vi "AE_AllStages_Action.vi"(6 "Velocity":dbl, 7 "Abort":refnum<vi>, 8 "Positions":dbl[](array[numeric]), 9 "Axis":bool[](array[boolean]), 10 "Stage ID":string, 11 "Action":T1=enum."MVR") -> (0 "Position Out":dbl[](array[numeric]), 1 "Status":bool, 2 "Special Function Out":string)   [LabVIEW 2014]
uses:
  Controls/StageStates.ctl
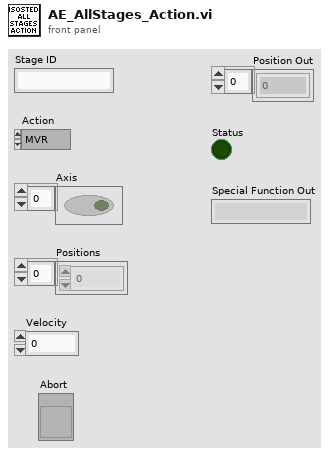
[diagram p1: front panel]
types:
  T1 = typedef "StageStates.ctl" = enum16{"POSITION", "MVR", "MOVE", "HALT", "ONTARGET", "ERROR", "EXIT", "HOME", "ZEROPOS", "NANOPOS", "QUIT", "ANALOG"}
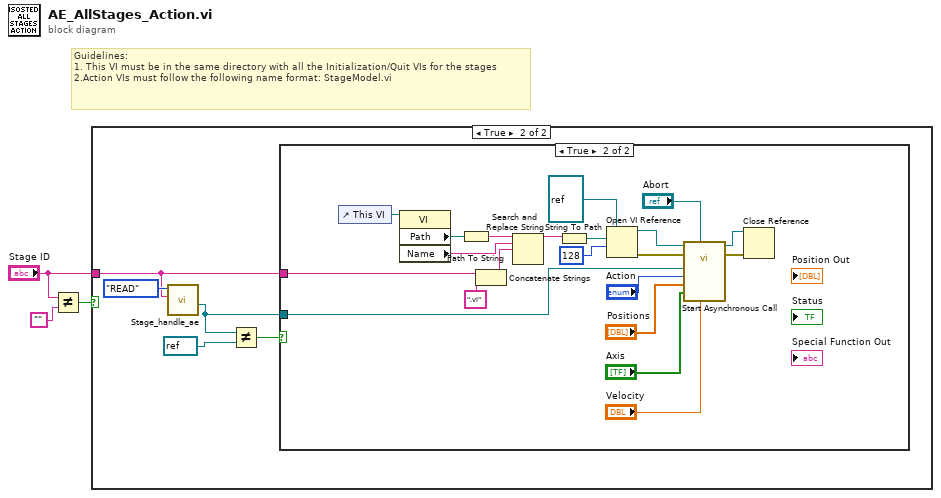
[diagram p0: block diagram]
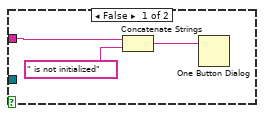
[diagram p3: hidden frame]
diagram:
  # "Guidelines:\n1. This VI must be in the same directory with all the Initialization/Quit VIs for the stages\n2.Action VIs must follow the following name format: StageModel.vi"
  n1 = Not Equal?(x="Stage ID", y="") -> (x != y?=w1:bool)
  n2 = case shown="True" w1 {
    tunnel: "Stage ID" -> [_ w4]
    frame False {
    }
    frame True {
      n3 = call "Stage_handle_ae.vi"("StageID"=w4, "Enum"=enum16{"WRITE", "READ"}."READ") -> ("Visa Out"=w5:refnum<visa-resource-name>)  [unwired: 9 in]
      n4 = Not Equal?(x=w5, y=refnum<visa-resource-name> refnum ("Visa Out")) -> (x != y?=w6:bool)
      n5 = case shown="True" w6 {
        tunnel: w4 -> [w11 w28]
        tunnel: w5 -> [_ w16]
        frame False {
          n6 = Concatenate Strings(w11, " is not initialized" ("string")) -> (w9:string)
          n7 = One Button Dialog(message=w9) -> ()  [unwired: 1 in, 1 out]
        }
        frame True {
          n8 = control-ref of="This VI"() -> (w32:refnum<vi>)
          n9 = property class="VI"(reference=w32) -> ("Path"=w31:path, "Name"=w29:string)  [unwired: 1 in, 2 out]
          n10 = Path To String(path=w31) -> (string=w30:string)
          n11 = Concatenate Strings(w28, ".vi" ("string")) -> (w21:string)
          n12 = Search and Replace String(input string=w30, search string=w29, replace string=w21) -> (result string=w27:string)  [unwired: 5 in, 3 out]
          n13 = String To Path(string=w27) -> (path=w26:path)
          n14 = Open VI Reference(type specifier VI Refnum (for type only)=refnum<vi> refnum, vi path=w26, options=128) -> (vi reference=w14:refnum<vi>, error out=w23:errorcluster)  [unwired: 3 in]
          n15 = call-by-ref "Start Asynchronous Call"(reference=w14, error in=w23, "Velocity"="Velocity", "Abort"="Abort", "Axis"="Axis", "Positions In"="Positions", "Action"="Action", "VISA In"=w16) -> (reference out=w24:refnum<vi>, error out=w22:errorcluster)  [unwired: 2 in, 4 out]
          n16 = Close Reference(reference=w24, error in (no error)=w22) -> ()  [unwired: 1 out]
        }
      }
    }
  }
